vi "NIIE_Icon Editor First Call.vi"(8 "error in (no error)":errorcluster) -> (0 "error out":errorcluster)   [LabVIEW 2021]
uses:
  <vilib>/picture/picture.llb/imagedata.ctl
  vi.lib/LabVIEW Icon API/lv_icon/Controls/Pathes.ctl
  <resource>/dialog/lvconfig.llb/LV Config Read Boolean.vi
  <resource>/dialog/lvconfig.llb/LV Config Write Boolean.vi
  vi.lib/LabVIEW Icon API/lv_icon/lv_icon.lvlib
panel:
  in  "Cluster 2":cluster{"path":path, "image data":T1}={"path"=path "Frameworks/_blank.png", "image data"={"image type"=0, "image depth"=24, "image"=array[3072 elements], "mask"=[], "colors"=[], "Rectangle"={"left"=0, "top"=0, "right"=32, "bottom"=32}}}
  in  "Cluster":cluster{"path":path, "image data":T1}={"path"=path "Frameworks/_blank.png", "image data"={"image type"=0, "image depth"=24, "image"=array[3072 elements], "mask"=[], "colors"=[], "Rectangle"={"left"=0, "top"=0, "right"=32, "bottom"=32}}}
  in  "String":string="_blank"
  in  "path":string="Frameworks"
  # "On Linux it is not possible to create the LabVIEW Data folder during the installation process.\nTherefore, this VI takes care to 'install' some glyphs and icon templates."
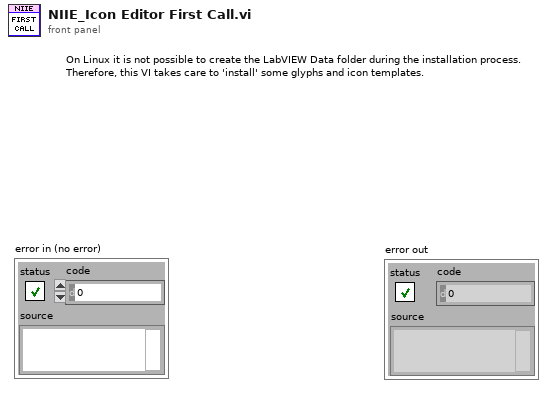
[diagram p1: front panel]
types:
  T1 = typedef "imagedata.ctl" = cluster{"image type":i32, "image depth":i32, "image":u8[], "mask":u8[], "colors":u32[], "Rectangle":cluster{"left":i16, "top":i16, "right":i16, "bottom":i16}}
  T2 = typedef "Pathes.ctl" = enum16{"Root Path", "Icon Templates", "Icon Templates VI", "Icon Templates Lib", "Glyphs"}
  T3 = cluster{"folder name":string, "file":string, "image data":T1}[]
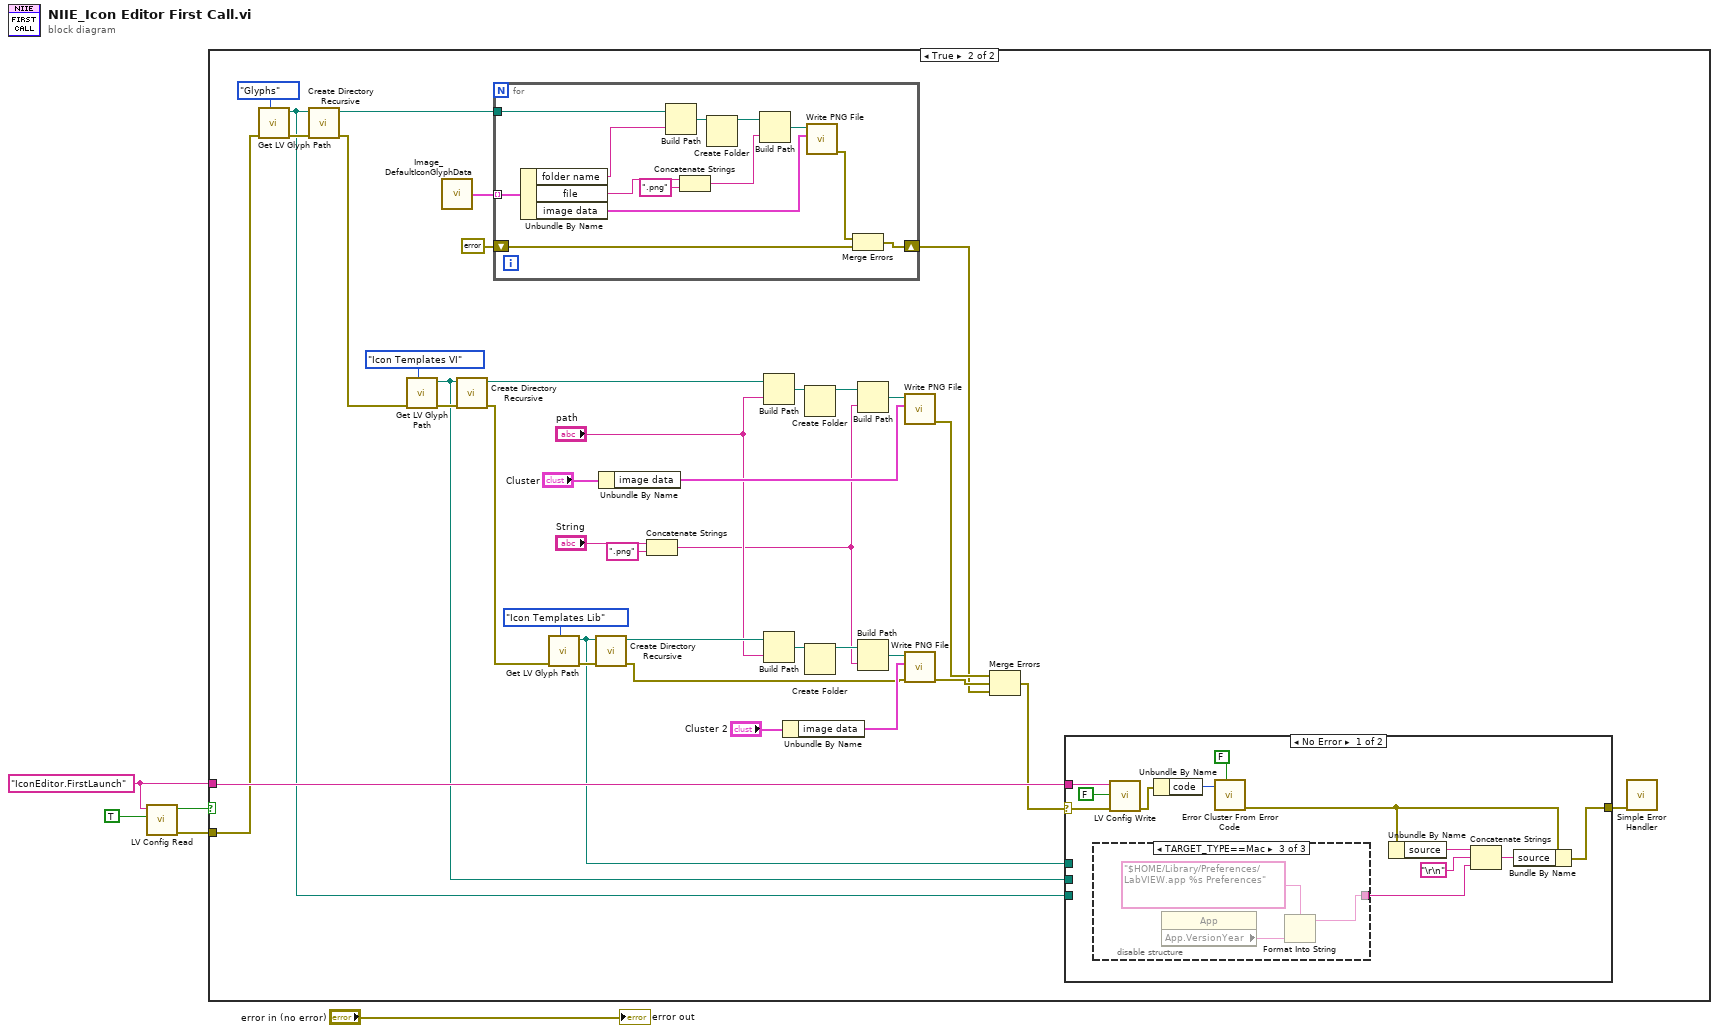
[diagram p0: block diagram]
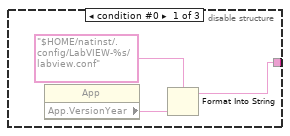
[diagram p3: hidden frame]
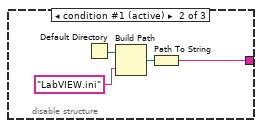
[diagram p4: hidden frame]
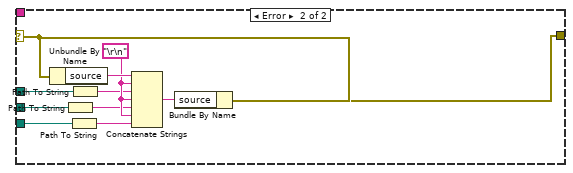
[diagram p5: hidden frame]
diagram:
  w3 = "IconEditor.FirstLaunch"
  n1 = call-poly <resource>:"LV Config Read.vi"("default value"=TRUE, "key"=w3) -> ("error out"=w4:errorcluster, "value"=w1:bool)  [unwired: 1 in, 3 out]
  n2 = case shown="True" w1 {
    tunnel: w4 -> [_ w8]
    tunnel: w3 -> [_ w40]
    frame False {
    }
    frame True {
      n3 = call "Get LV Glyph Path.vi"("Path"=Pathes."Glyphs", "error in (no error)"=w8) -> ("error out"=w35:errorcluster, "Requested Path"=w9:path)  [unwired: 1 in, 7 out]
      n4 = call <vilib>:"Create Directory Recursive.vi"("error in (no error)"=w35, "directory"=w9) -> ("error out"=w14:errorcluster, "directory copy"=w34:path)  [unwired: 1 in, 3 out]
      n5 = call "Get LV Glyph Path.vi"("Path"=Pathes."Icon Templates VI", "error in (no error)"=w14) -> ("error out"=w39:errorcluster, "Requested Path"=w10:path)  [unwired: 1 in, 7 out]
      n6 = call "Image_DefaultIconGlyphData.vi"() -> ("defaultImageInfo"=w6:T3)  [unwired: 1 in]
      n7 = call <vilib>:"Create Directory Recursive.vi"("error in (no error)"=w39, "directory"=w10) -> ("error out"=w13:errorcluster, "directory copy"=w38:path)  [unwired: 1 in, 3 out]
      n8 = for {
        tunnel: w34 -> [w89]
        tunnel: w6 -> [w87] mode=indexing
        shift-right: [w78] -> w15
        shift-left: errorcluster {"status"=FALSE, "code"=0, "source"=""} ("error IO") -> [w77]
        n9 = Unbundle By Name(w87) -> ("folder name"=w83:string, "file"=w82:string, "image data"=w84:T1)
        n10 = Build Path(base path=w89, name or relative path=w83) -> (appended path=w88:path)
        n11 = Concatenate Strings(w82, ".png" ("string")) -> (w80:string)
        n12 = Create Folder(path (use dialog)=w88) -> (created path=w86:path)  [unwired: 2 in, 2 out]
        n13 = Build Path(base path=w86, name or relative path=w80) -> (appended path=w85:path)
        n14 = call <vilib>:"Write PNG File.vi"("image data"=w84, "path to PNG file"=w85) -> ("error out"=w79:errorcluster)  [unwired: 2 in, 7 out]
        n15 = Merge Errors(w79, w77) -> (w78:errorcluster)
      }
      n16 = call "Get LV Glyph Path.vi"("Path"=Pathes."Icon Templates Lib", "error in (no error)"=w13) -> ("error out"=w37:errorcluster, "Requested Path"=w11:path)  [unwired: 1 in, 7 out]
      n17 = call <vilib>:"Create Directory Recursive.vi"("error in (no error)"=w37, "directory"=w11) -> ("error out"=w12:errorcluster, "directory copy"=w36:path)  [unwired: 1 in, 3 out]
      n18 = Unbundle By Name("Cluster") -> ("image data"=w30:T1)
      n19 = Concatenate Strings("String", ".png" ("string")) -> (w18:string)
      n20 = Build Path(base path=w38, name or relative path="path") -> (appended path=w33:path)
      n21 = Build Path(base path=w36, name or relative path="path") -> (appended path=w28:path)
      n22 = Unbundle By Name("Cluster 2") -> ("image data"=w25:T1)
      n23 = Create Folder(path (use dialog)=w33) -> (created path=w32:path)  [unwired: 2 in, 2 out]
      n24 = Create Folder(path (use dialog)=w28) -> (created path=w27:path)  [unwired: 2 in, 2 out]
      n25 = Build Path(base path=w32, name or relative path=w18) -> (appended path=w31:path)
      n26 = Build Path(base path=w27, name or relative path=w18) -> (appended path=w26:path)
      n27 = call <vilib>:"Write PNG File.vi"("image data"=w30, "path to PNG file"=w31) -> ("error out"=w22:errorcluster)  [unwired: 2 in, 7 out]
      n28 = call <vilib>:"Write PNG File.vi"("error in (no error)"=w12, "image data"=w25, "path to PNG file"=w26) -> ("error out"=w23:errorcluster)  [unwired: 1 in, 7 out]
      n29 = Merge Errors(w22, w23, w15) -> (w16:errorcluster)
      n30 = case shown="No Error" w16 {
        selector: w16 -> [w45 w74]
        tunnel: w40 -> [w54 _]
        tunnel: [w46 w66] -> w17
        tunnel: w11 -> [_ w72]
        tunnel: w10 -> [_ w70]
        tunnel: w9 -> [_ w68]
        frame No Error {
          n31 = disable-structure shown="TARGET_TYPE==Mac" {
            disable-tunnel: [w56 w59 w63] -> w44
            frame condition #0 {
              n32 = property class="App"() -> ("App.VersionYear"=w57:string)  [unwired: 2 in, 2 out]
              n33 = Format Into String(format string="$HOME/natinst/.config/LabVIEW-%s/labview.conf" ("name or relative path"), w57) -> (resulting string=w56:string)  [unwired: 2 in, 1 out]
            }
            frame condition #1 (active) {
              n34 = Default Directory() -> (w61:path)
              n35 = Build Path(base path=w61, name or relative path="LabVIEW.ini") -> (appended path=w62:path)
              n36 = Path To String(path=w62) -> (string=w59:string)
            }
            frame condition #2 {
              n37 = property class="App"() -> ("App.VersionYear"=w64:string)  [unwired: 2 in, 2 out]
              n38 = Format Into String(format string="$HOME/Library/Preferences/LabVIEW.app %s Preferences" ("name or relative path"), w64) -> (resulting string=w63:string)  [unwired: 2 in, 1 out]
            }
          }
          n39 = call-poly <resource>:"LV Config Write.vi"("error in (no error)"=w45, "value"=FALSE, "key"=w54) -> ("error out"=w52:errorcluster)  [unwired: 4 out]
          n40 = Unbundle By Name(w52) -> ("code"=w51:i32)
          n41 = call <vilib>:"Error Cluster From Error Code.vi"("show call chain? (False)"=FALSE, "error code (0)"=w51) -> ("error out"=w48:errorcluster)  [unwired: 7 in]
          n42 = Unbundle By Name(w48) -> ("source"=w50:string)
          n43 = Concatenate Strings(w50, "\r\n", w44) -> (w47:string)
          n44 = Bundle By Name(cluster=w48, "source"=w47) -> (w46:errorcluster)
        }
        frame Error {
          w73 = "\r\n"
          n45 = Unbundle By Name(w74) -> ("source"=w76:string)
          n46 = Path To String(path=w70) -> (string=w69:string)
          n47 = Path To String(path=w68) -> (string=w67:string)
          n48 = Path To String(path=w72) -> (string=w71:string)
          n49 = Concatenate Strings(w76, w73, w71, w73, w69, w73, w67) -> (w75:string)
          n50 = Bundle By Name(cluster=w74, "source"=w75) -> (w66:errorcluster)
        }
      }
      n51 = call <vilib>:"Simple Error Handler.vi"("error in (no error)"=w17) -> ()  [unwired: 4 in, 5 out]
    }
  }
  "error out" <- "error in (no error)"
